vi "Format data to plot.vi"(8 "Data Array 2":dbl[][](array[numeric]), 11 "Data Array":dbl[][](array[numeric])) -> (3 "JV Curve":cluster{"Y":dbl[], "Y":dbl[]}[](graph))   [LabVIEW 2011]
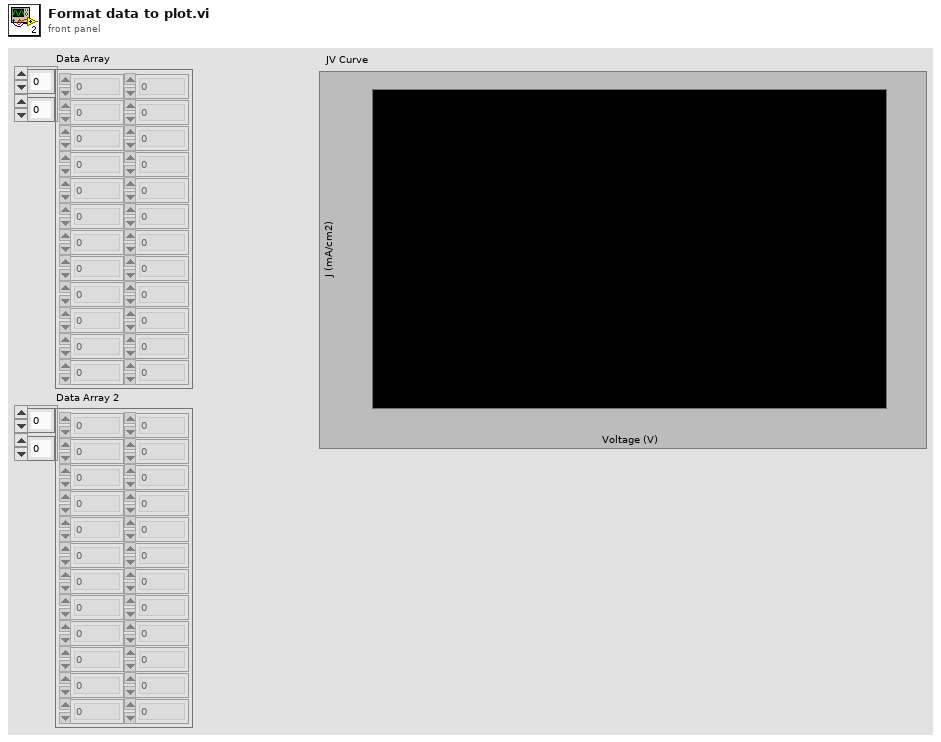
[diagram p1: front panel]
types:
  T1 = cluster{"Data Array 2":dbl[], "Data Array 2":dbl[]}
  T2 = cluster{"Data Array 2":dbl[], "Data Array 2":dbl[]}[]
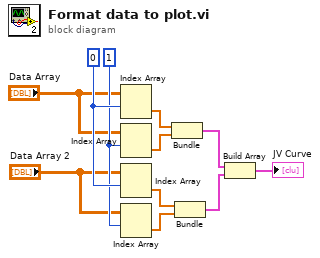
[diagram p0: block diagram]
diagram:
  w10 = 1
  w11 = 0
  n1 = Index Array(array="Data Array", index (row)=w11) -> (element=w7:dbl[])  [unwired: 1 in]
  n2 = Index Array(array="Data Array", index (row)=w10) -> (element=w6:dbl[])  [unwired: 1 in]
  n3 = Index Array(array="Data Array 2", index (row)=w11) -> (element=w5:dbl[])  [unwired: 1 in]
  n4 = Index Array(array="Data Array 2", index (row)=w10) -> (element=w4:dbl[])  [unwired: 1 in]
  n5 = Bundle("Data Array"=w7, "Data Array"=w6) -> (w2:cluster{"Data Array":dbl[], "Data Array":dbl[]})  [unwired: 1 in]
  n6 = Bundle("Data Array 2"=w5, "Data Array 2"=w4) -> (w3:T1)  [unwired: 1 in]
  n7 = Build Array(w2, w3) -> (→"JV Curve":T2)
